vi "Write RT hardware channels.vi"(8 "error in":errorcluster, 10 "RT hardware channels":T1[](array[typedef]) {"labels settings for RT"."Label Timestamp Channel Data Reference" format="%.0x"; "labels settings for RT"."Word Initial Raw Value" format="%032.0f"; "labels settings for RT"."Label Disable/Trigger Channel Reference" format="%.0x"; "labels settings for RT"."parameter driver data"."Tx parameter refs" format="%.0x"; "labels settings for RT"."SDI" format="%02b"; "labels settings for RT"."label" format="%.0o"}, 11 "Rx execution unit in":refnum<class "Rx Execution Unit.lvclass">) -> (0 "error out":errorcluster, 3 "Rx execution unit out":refnum<class "Rx Execution Unit.lvclass">)   [LabVIEW 2020, in "AIM ARINC 429 Engine.lvlib" / "Implementation.lvlib" / "Rx Execution Unit.lvclass"]
uses:
  Rx Execution Unit.lvclass
  Shared/RT Hardware Channel Settings.ctl
  Shared/RT Label Settings.ctl
  Shared/Label.ctl
  Shared/RT Parameters.ctl
  Shared/Parameter Definition.ctl
  <vilib>/NI/NI VeriStand Encoding and Decoding/Encoding.ctl
  <vilib>/NI VeriStand/Custom Device API/Custom Device Item Ref.ctl
  Shared/Transfer Type.ctl
  <vilib>/NI VeriStand/Custom Device API/Data Reference.ctl
  Rx Execution Unit.lvclass/Rx Execution Unit.ctl
  <vilib>/NI/NI VeriStand Encoding and Decoding/Encoding and Decoding.lvlib
  <vilib>/NI VeriStand/Custom Device API/Custom Device API.lvlib
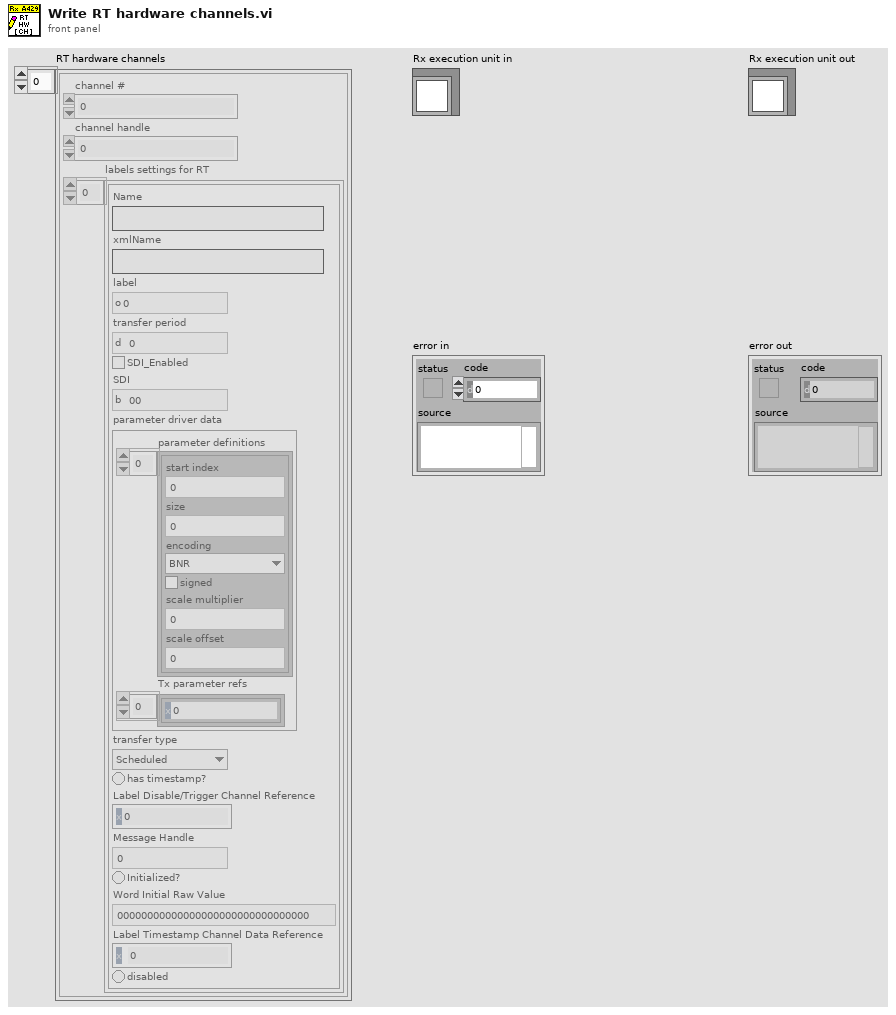
[diagram p1: front panel]
types:
  T1 = typedef "RT Hardware Channel Settings.ctl" = cluster{"channel #":u16, "channel handle":u64, "labels settings for RT":T2[]}
  T2 = typedef "RT Label Settings.ctl" = cluster{"Name":string, "xmlName":string, "label":T3, "transfer period":u32, "SDI_Enabled":bool, "SDI":u8, "parameter driver data":T4, "transfer type":T8, "has timestamp?":bool, "Label Disable/Trigger Channel Reference":T7, "Message Handle":u64, "Initialized?":bool, "Word Initial Raw Value":u32, "Label Timestamp Channel Data Reference":T9, "disabled":bool}
  T3 = typedef "Label.ctl" = u8
  T4 = typedef "RT Parameters.ctl" = cluster{"parameter definitions":T5[], "Tx parameter refs":T7[]}
  T5 = typedef "Parameter Definition.ctl" = cluster{"start index":i32, "size":i32, "encoding":T6, "signed":bool, "scale multiplier":dbl, "scale offset":dbl}
  T6 = typedef "Encoding and Decoding.lvlib/Encoding.ctl" = enum16{"BNR", "BCD", "Discrete"}
  T7 = typedef "Custom Device API.lvlib/Custom Device Item Ref.ctl" = u64
  T8 = typedef "Transfer Type.ctl" = enum16{"Scheduled", "Acyclic", "Block", "Strobe"}
  T9 = typedef "Custom Device API.lvlib/Data Reference.ctl" = i32
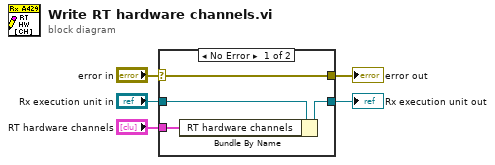
[diagram p0: block diagram]
diagram:
  n1 = case shown="No Error" "error in" {
    selector: "error in" -> [w9 w10]
    tunnel: [w9 w10] -> w4
    tunnel: [w7 w11] -> w2
    tunnel: "Rx execution unit in" -> [w8 w11]
    tunnel: "RT hardware channels" -> [w6 _]
    frame No Error {
      n2 = Bundle By Name(cluster=w8, "RT hardware channels"=w6) -> (w7:refnum<class "Rx Execution Unit.lvclass">)
    }
    frame Error {
    }
  }
  "error out" <- w4
  "Rx execution unit out" <- w2
